vi "关闭.vi"(8 "error in (no error)":errorcluster caption="错误输入（无错误）", 11 "通讯类 输入":refnum<class "通讯类.lvclass">) -> (0 "error out":errorcluster caption="错误输出")   [LabVIEW 2016, in "通讯类.lvclass"]
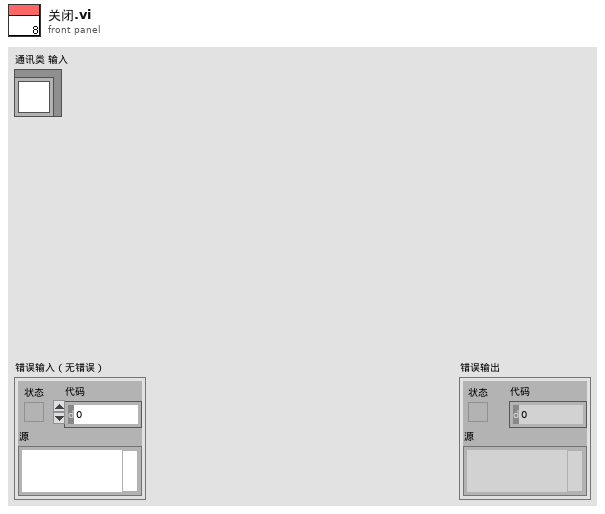
[diagram p1: front panel]
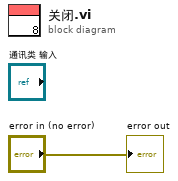
[diagram p0: block diagram]
diagram:
  "error out" <- "error in (no error)"
